vi "UTILITY Simple PID.vi"(4 "Use Proportion Valve":bool, 6 "K(0.1)":dbl=0.3, 8 "Error In":errorcluster, 9 "GPM Target(3)":dbl, 10 "GPM reading":dbl, 11 "Previous MicroAmp":dbl) -> (0 "Error Out":errorcluster, 2 "Adjustment Factor":dbl, 3 "New MicroAmp":dbl)   [LabVIEW 2018]
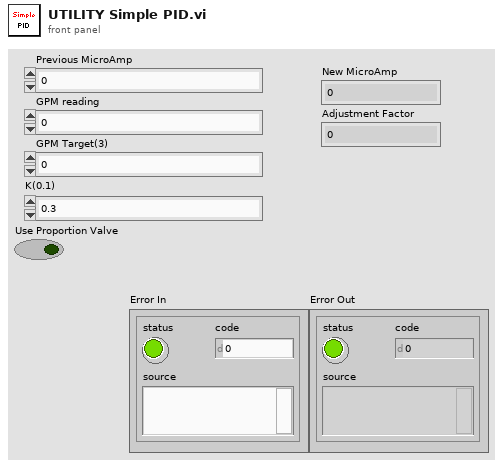
[diagram p1: front panel]
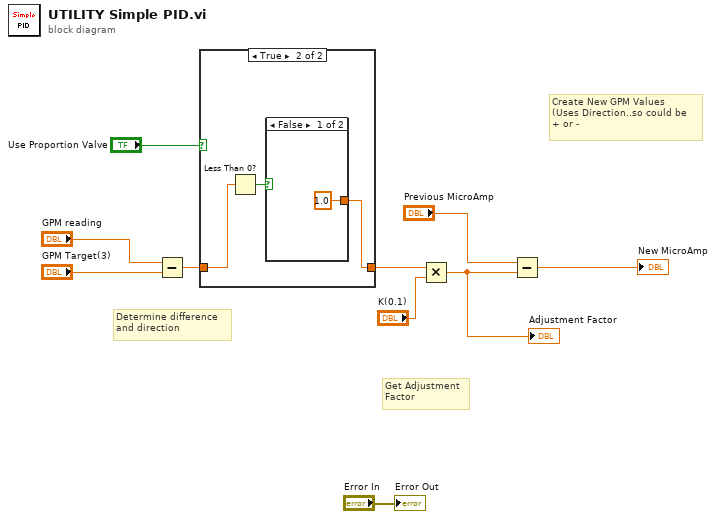
[diagram p0: block diagram]
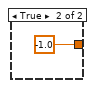
[diagram p3: hidden frame]
diagram:
  # "Create New GPM Values\n(Uses Direction..so could be \n+ or -"
  # "Get Adjustment\nFactor"
  # "Determine difference \nand direction"
  n1 = Subtract(x="GPM reading", y="GPM Target(3)") -> (x-y=w2:dbl)
  n2 = case shown="True" "Use Proportion Valve" {
    tunnel: w2 -> [w11 w14]
    tunnel: [w11 w12] -> w1
    frame False {
    }
    frame True {
      n3 = Less Than 0?(x=w14) -> (x < 0?=w13:bool)
      n4 = case shown="False" w13 {
        tunnel: [1.0 -1.0] -> w12
        frame False {
        }
        frame True {
        }
      }
    }
  }
  n5 = Multiply(x=w1, y="K(0.1)") -> (x*y=w6:dbl)
  "Adjustment Factor" <- w6
  n6 = Subtract(x="Previous MicroAmp", y=w6) -> (x-y=→"New MicroAmp":dbl)
  "Error Out" <- "Error In"
